vi "Create.vi"(8 "error in (no error)":errorcluster, 10 "Sequence Context In":refnum<k7>) -> (0 "error out":errorcluster, 3 "TSContext Configuration":refnum<class "TSContext Configuration.lvclass">)   [LabVIEW 2020, in "Astemes_CSVReportPlugin.lvlib" / "TSContext Configuration.lvclass"]
uses:
  TSContext Configuration.lvclass
  TSContext Configuration.lvclass/TSContext Configuration.ctl
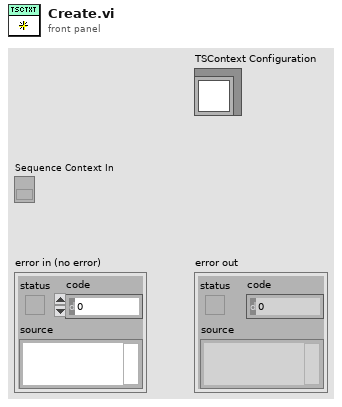
[diagram p1: front panel]
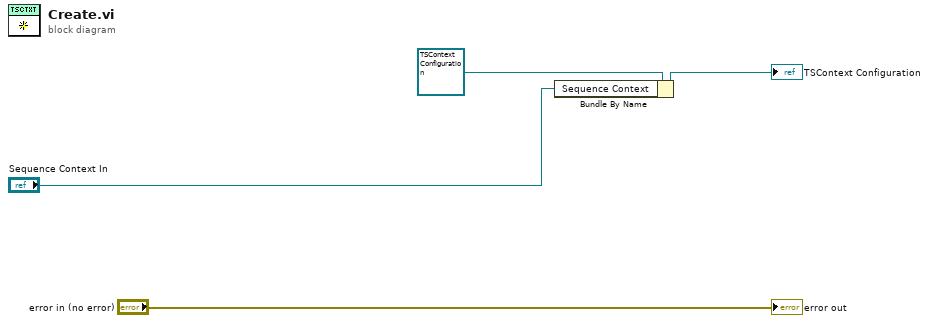
[diagram p0: block diagram]
diagram:
  n1 = Bundle By Name(cluster=refnum<class "TSContext Configuration.lvclass"> refnum ("TSContext Configuration"), "Sequence Context"="Sequence Context In") -> (→"TSContext Configuration":refnum<class "TSContext Configuration.lvclass">)
  "error out" <- "error in (no error)"
